vi "Get Next Move.vi"(8 "error in (no error)":errorcluster caption="entrée d'erreur (pas d'erreur)", 10 "Move queue":refnum<queue>, 11 "Game Board en entrée":refnum<class "Game Board.lvclass">) -> (0 "error out":errorcluster caption="sortie d'erreur", 2 "Freeze Piece":bool, 3 "Game Board en sortie":refnum<class "Game Board.lvclass">)   [LabVIEW 2017, in "Game Board.lvclass"]
uses:
  Game Board.lvclass
  Controls/Moves.ctl
  Controls/Coordinates.ctl
  Game Board.lvclass/Game Board.ctl
  Wall_class/Wall.lvclass
  Piece of Bricks_class/Piece of Bricks.lvclass
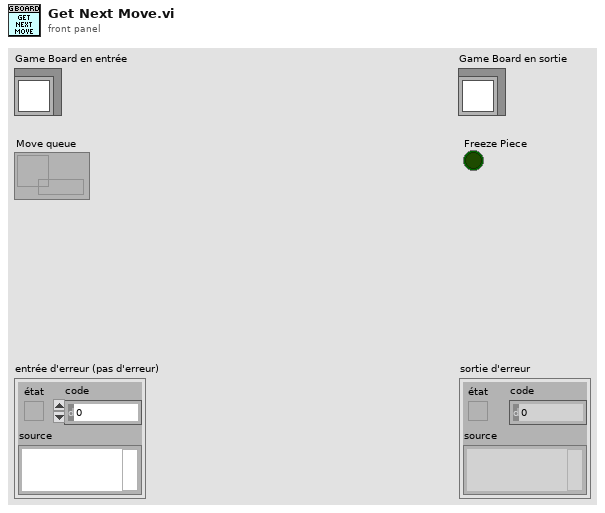
[diagram p1: front panel]
types:
  T1 = typedef "Coordinates.ctl" = cluster{"X":i32, "Y":i32}
  T2 = typedef "Moves.ctl" = enum16{"None", "Right", "Left", "Step Down", "Go Down", "90 Clockwise", "90 Anti-Clockwise"}
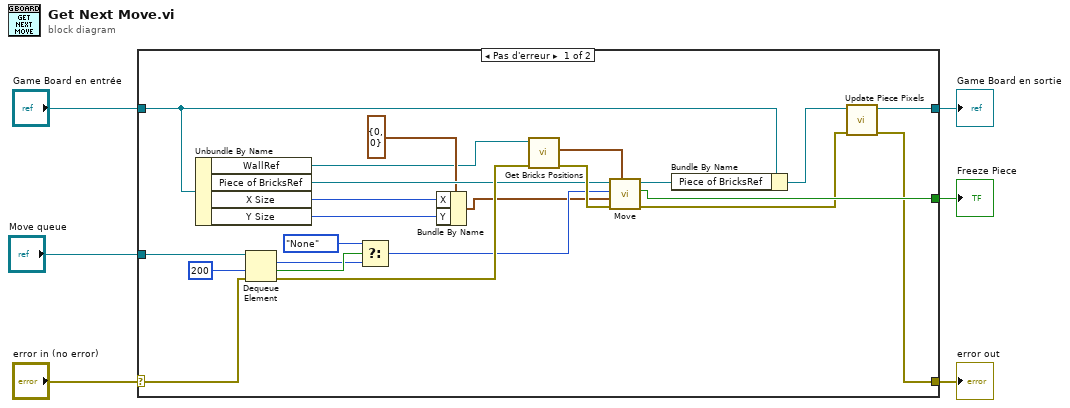
[diagram p0: block diagram]
diagram:
  n1 = case shown="Pas d'erreur" "error in (no error)" {
    selector: "error in (no error)" -> [w24 w31]
    tunnel: [w9 w31] -> w5
    tunnel: [w11 w30] -> w3
    tunnel: "Game Board en entrée" -> [w27 w30]
    tunnel: "Move queue" -> [w23 _]
    tunnel: [w13 _] -> w1
    frame No Error {
      n2 = Unbundle By Name(w27) -> ("WallRef"=w15:refnum<class "Wall.lvclass">, "Piece of BricksRef"=w26:refnum<class "Piece of Bricks.lvclass">, "X Size"=w8:i32, "Y Size"=w7:i32)
      n3 = Dequeue Element(queue=w23, timeout in ms (-1)=200 ("timeout en ms (-1)"), error in (no error)=w24) -> (element=w21:T2, timed out?=w22:bool, error out=w29:errorcluster)  [unwired: 1 out]
      n4 = Select(t=Moves."None" ("cas vrai"), s=w22, f=w21) -> (s? t:f=w20:T2)
      n5 = Bundle By Name(cluster=T1 {"X"=0, "Y"=0} ("Coordinates"), "X"=w8, "Y"=w7) -> (w16:T1)
      n6 = call-dynamic "Get Bricks Positions.vi"("error in (no error)"=w29, "object in"=w15) -> ("error out"=w28:errorcluster, "Brick Wall"=w14:T1[])  [unwired: 7 in, 1 out]
      n7 = call-dynamic "Move.vi"("Wall Positions"=w14, "error in (no error)"=w28, "GameBoard Size"=w16, "Move"=w20, "object in"=w26) -> ("error out"=w10:errorcluster, "Freeze Piece"=w13:bool, "object out"=w25:refnum<class "Piece of Bricks.lvclass">)  [unwired: 4 in]
      n8 = Bundle By Name(cluster=w27, "Piece of BricksRef"=w25) -> (w12:refnum<class "Game Board.lvclass">)
      n9 = call-dynamic "Update Piece Pixels.vi"("error in (no error)"=w10, "Game Board en entrée"=w12) -> ("error out"=w9:errorcluster, "Game Board en sortie"=w11:refnum<class "Game Board.lvclass">)  [unwired: 8 in]
    }
    frame Error {
    }
  }
  "error out" <- w5
  "Game Board en sortie" <- w3
  "Freeze Piece" <- w1
